vi "Generate a Message.vi"(8 "error in (no error)":errorcluster, 9 "Value":string, 10 "Keyword":string, 11 "Section":string) -> (0 "error out":errorcluster, 3 "Message":string)   [LabVIEW 2021, in "CANOpen Addon System Explorer.lvlib"]
uses:
  CANOpen Addon System Explorer.lvlib
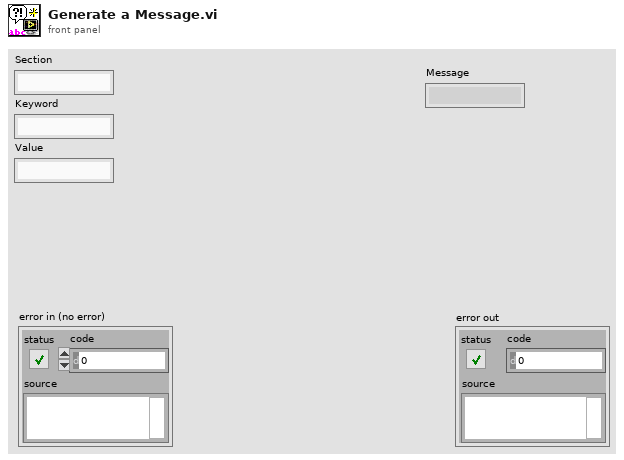
[diagram p1: front panel]
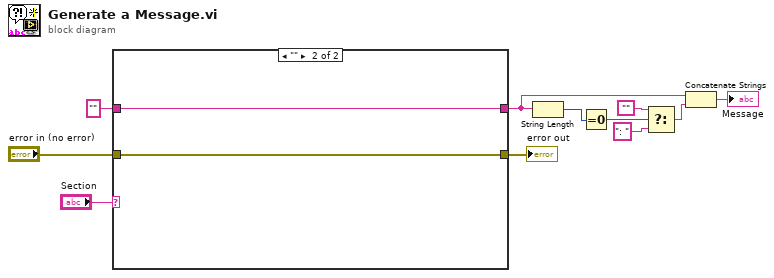
[diagram p0: block diagram]
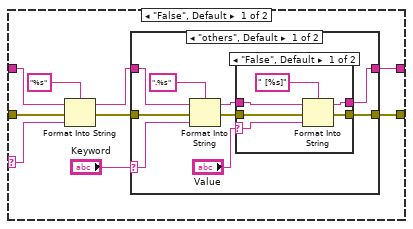
[diagram p2: hidden frame]
diagram:
  n1 = case shown="\"\"" "Section" {
    selector: "Section" -> [w18 _]
    tunnel: [w14 w41] -> w7
    tunnel: "" -> [w20 w41]
    tunnel: "error in (no error)" -> [w17 w40]
    tunnel: [w12 w40] -> w8
    frame "False", Default {
      n2 = Format Into String(format string="%s", initial string=w20, error in=w17, w18) -> (resulting string=w15:string, error out=w13:errorcluster)
      n3 = case shown="\"others\", Default" "Keyword" {
        selector: "Keyword" -> [w27 _]
        tunnel: w15 -> [w29 w39]
        tunnel: [w21 w39] -> w14
        tunnel: [w22 w38] -> w12
        tunnel: w13 -> [w28 w38]
        frame "others", Default {
          n4 = Format Into String(format string=".%s", initial string=w29, error in=w28, w27) -> (resulting string=w24:string, error out=w23:errorcluster)
          n5 = case shown="\"False\", Default" "Value" {
            selector: "Value" -> [w33 _]
            tunnel: w24 -> [w35 w36]
            tunnel: w23 -> [w34 w37]
            tunnel: [w30 w37] -> w22
            tunnel: [w31 w36] -> w21
            frame "False", Default {
              n6 = Format Into String(format string=" [%s]", initial string=w35, error in=w34, w33) -> (resulting string=w31:string, error out=w30:errorcluster)
            }
            frame "" {
            }
          }
        }
        frame "" {
        }
      }
    }
    frame "" {
    }
  }
  "error out" <- w8
  n7 = String Length(string=w7) -> (length=w6:i32)
  n8 = Equal To 0?(x=w6) -> (x = 0?=w5:bool)
  n9 = Select(t="", s=w5, f=": ") -> (s? t:f=w4:string)
  n10 = Concatenate Strings(w7, w4) -> (→"Message":string)
